vi "Resize Image to a Container 2012 NIVerified.vi"(7 "error in (no error)":errorcluster, 9 "image data":T1, 10 "Path to Image (PNG, JPEG, BMP)":path) -> (0 "error out":errorcluster, 3 "Resized Image":picture)   [LabVIEW 2021, in "Component Tray.lvclass"]
doc: "Demonstrate how to use Base LabVIEW functions and property nodes to manipulate different picture images"
uses:
  Component Tray.lvclass
  <vilib>/picture/picture.llb/imagedata.ctl
panel:
  out "Resized Container":picture
  out "Original":picture
  # "Overview：Demonstrate  how to use Base LabVIEW functions and property nodes to manipulate different picture images\nRequirements:  LabVIEW 2012 or compatible\nInstructions:\n1. Run the VI\n2. Select the location of the image file using the Path to Image control\n3. Run the VI"
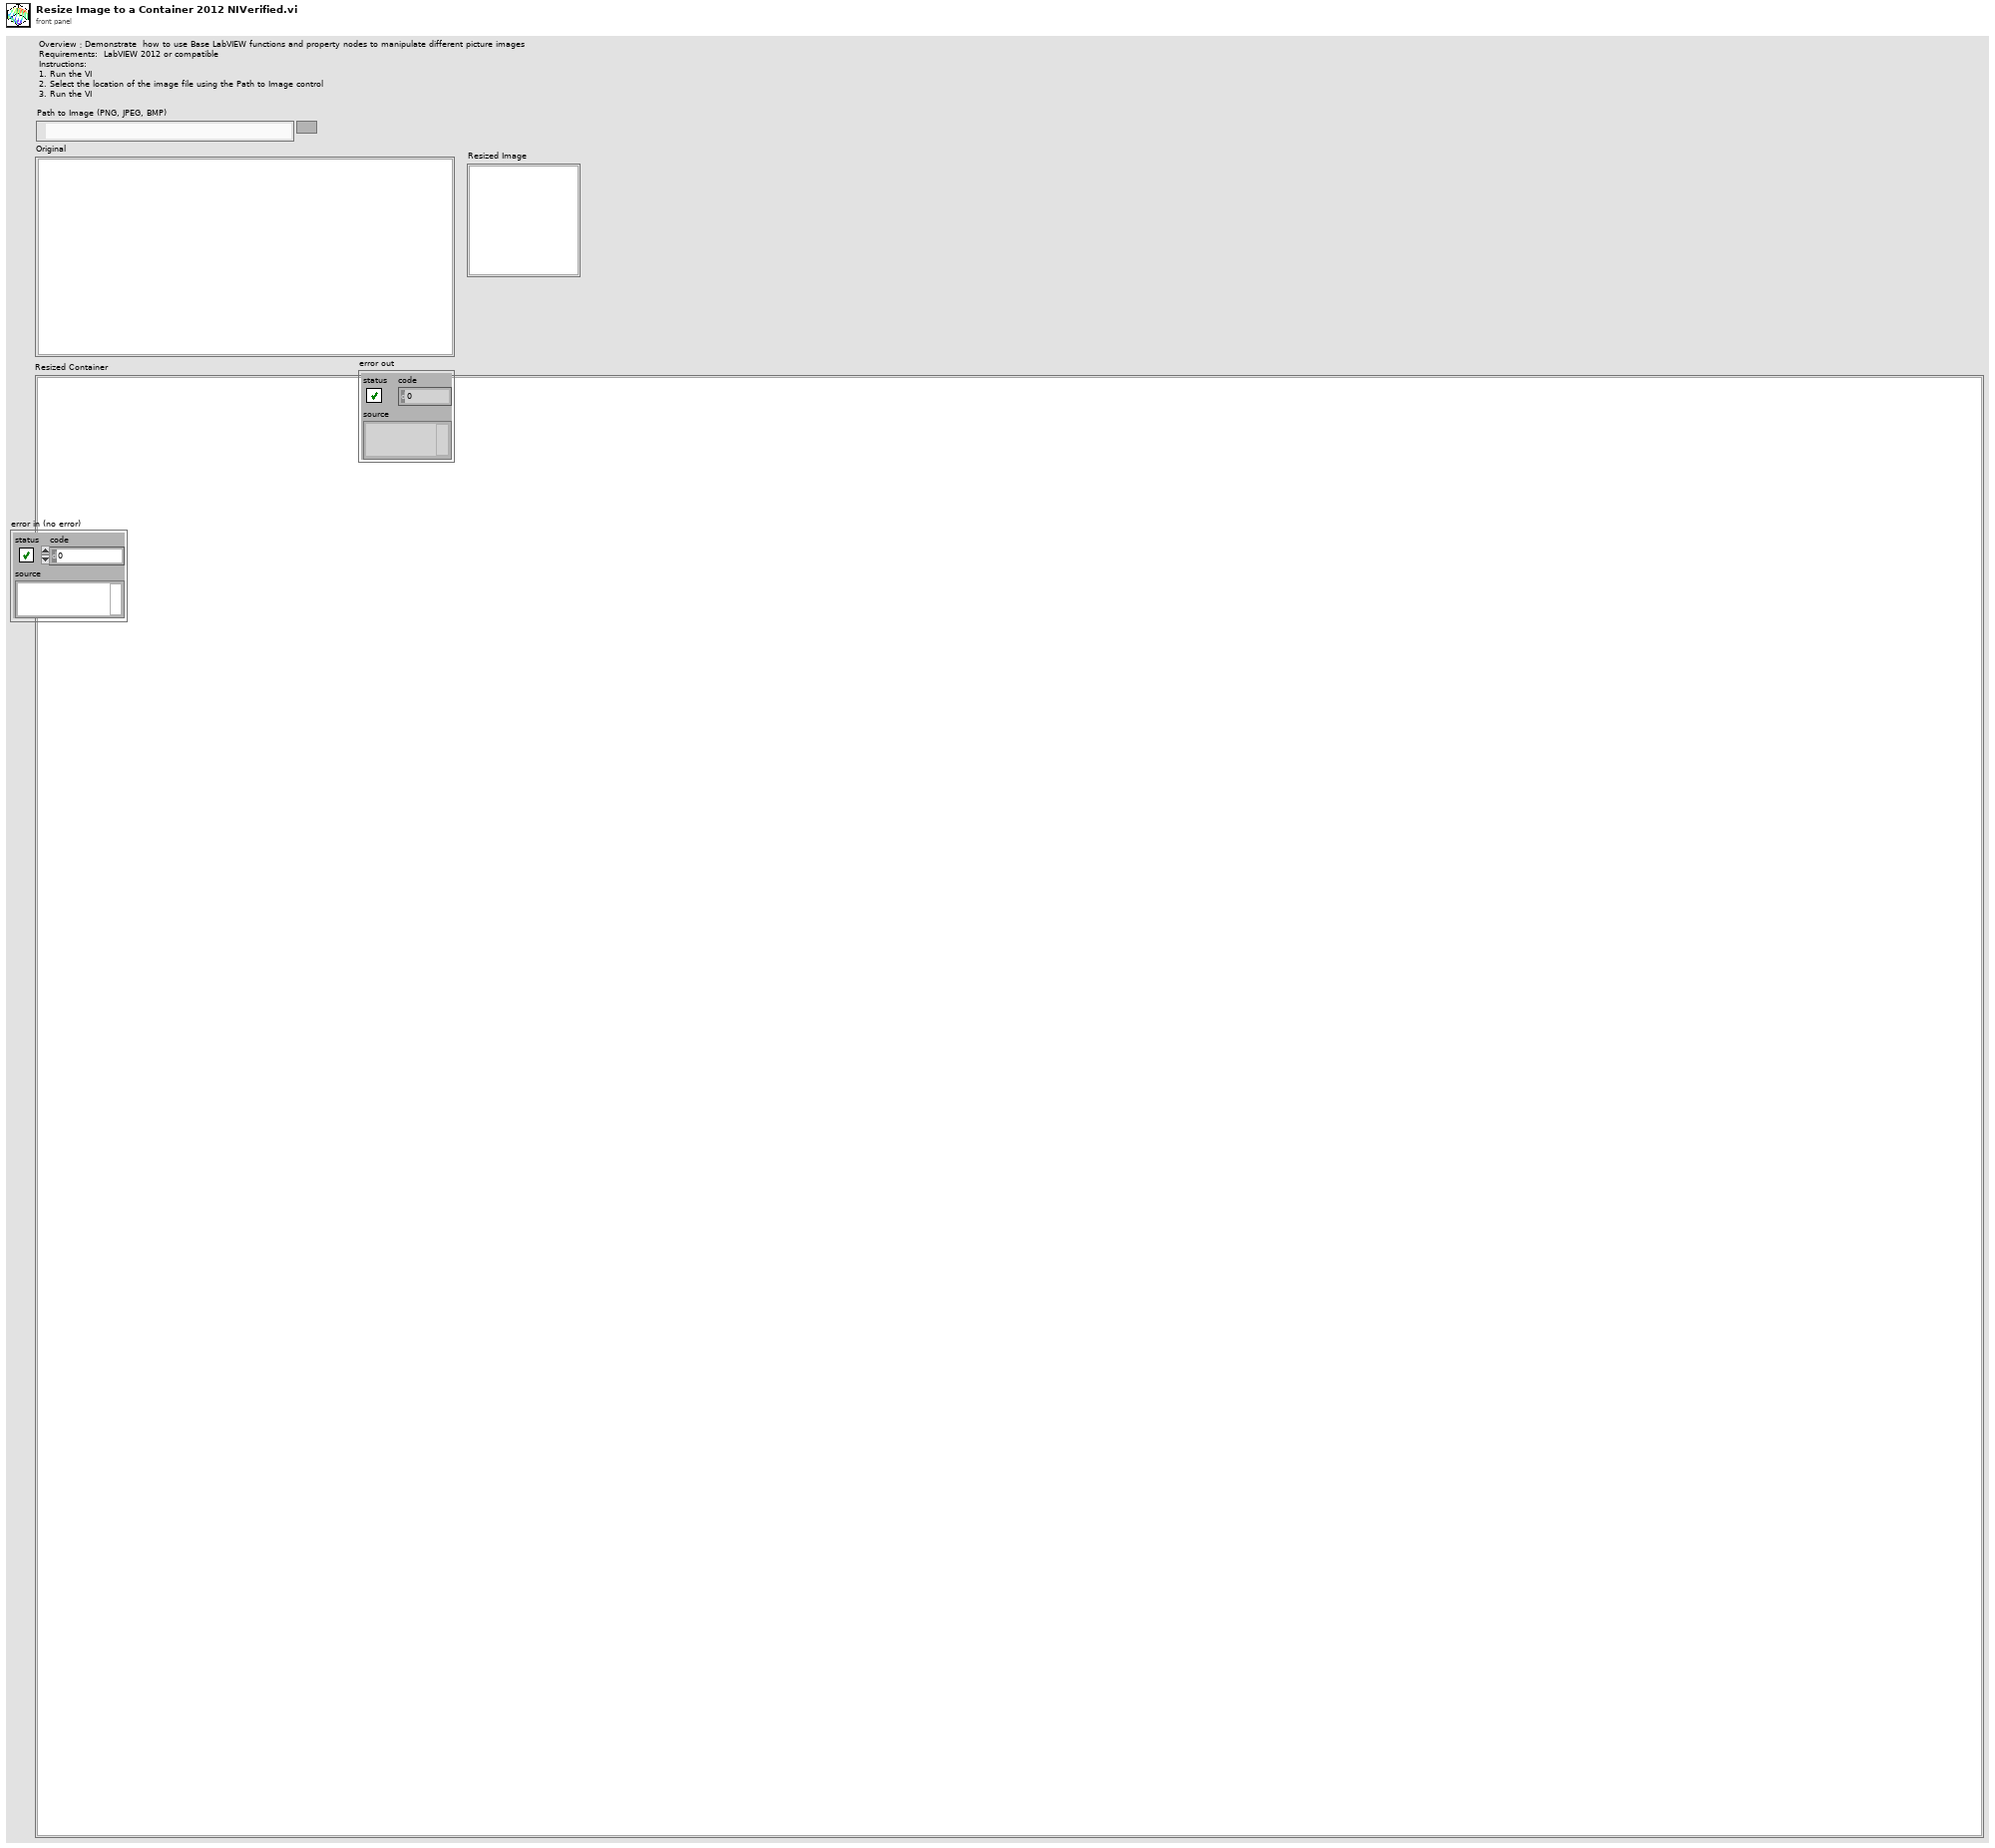
[diagram p1: front panel]
types:
  T1 = typedef "imagedata.ctl" = cluster{"image type":i32, "image depth":i32, "image":u8[], "mask":u8[], "colors":u32[], "Rectangle":cluster{"left":i16, "top":i16, "right":i16, "bottom":i16}}
  T2 = typedef "LVBoundsTypeDef.ctl" = cluster{"Width":u32, "Height":u32}
  T3 = cluster{"left":i16, "top":i16, "right":i16, "bottom":i16}
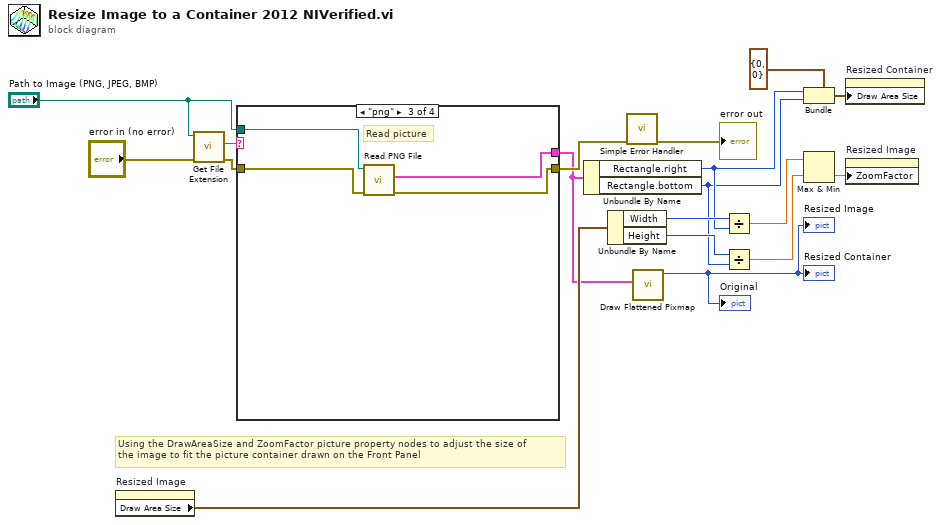
[diagram p0: block diagram]
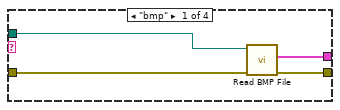
[diagram p2: hidden frame]
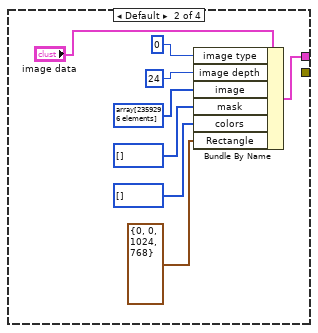
[diagram p3: hidden frame]
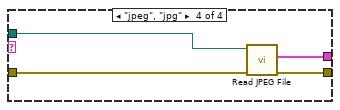
[diagram p4: hidden frame]
diagram:
  # "Using the DrawAreaSize and ZoomFactor picture property nodes to adjust the size of \nthe image to fit the picture container drawn on the Front Panel"
  n1 = property on="Resized Image" class="Pict"() -> ("Draw Area Size"=w18:T2)  [unwired: 2 in, 2 out]
  n2 = call <vilib>:"Get File Extension.vi"("error in (no error)"="error in (no error)", "file"="Path to Image (PNG, JPEG, BMP)") -> ("error out"=w5:errorcluster, "lowercase file extension"=w6:string)  [unwired: 5 in, 3 out]
  n3 = case shown="\"png\"" w6 {
    tunnel: "Path to Image (PNG, JPEG, BMP)" -> [w22 _ w34 w38]
    tunnel: [w21 w23 w33 w37] -> w3
    tunnel: [w20 _ w32 w36] -> w4
    tunnel: w5 -> [w19 _ w31 w35]
    frame "bmp" {
      n4 = call <vilib>:"Read BMP File.vi"("error in (no error)"=w19, "path to BMP file"=w22) -> ("error out"=w20:errorcluster, "image data"=w21:T1)  [unwired: 7 in, 1 out]
    }
    frame Default {
      n5 = Bundle By Name(cluster="image data", "image type"=0, "image depth"=24, "image"=u8[] array[2359296 elements], "mask"=u8[] [], "colors"=u32[] [], "Rectangle"=T3 {"left"=0, "top"=0, "right"=1024, "bottom"=768}) -> (w23:T1)
    }
    frame "png" {
      # "Read picture"
      n6 = call <vilib>:"Read PNG File.vi"("error in (no error)"=w31, "path to PNG file"=w34) -> ("error out"=w32:errorcluster, "image data"=w33:T1)  [unwired: 7 in, 1 out]
    }
    frame "jpeg", "jpg" {
      n7 = call <vilib>:"Read JPEG File.vi"("error in (no error)"=w35, "path to JPEG file"=w38) -> ("error out"=w36:errorcluster, "image data"=w37:T1)  [unwired: 7 in, 1 out]
    }
  }
  n8 = Unbundle By Name(w3) -> ("Rectangle.right"=w12:i16, "Rectangle.bottom"=w11:i16)
  n9 = Unbundle By Name(w18) -> ("Width"=w17:u32, "Height"=w16:u32)
  n10 = call <vilib>:"Simple Error Handler.vi"("error in (no error)"=w4) -> ("error out"=→"error out":errorcluster)  [unwired: 4 in, 4 out]
  n11 = call <vilib>:"Draw Flattened Pixmap.vi"("image data"=w3) -> ("new picture"=→"Resized Image" →"Original" →"Resized Container":picture)  [unwired: 8 in]
  n12 = Divide(x=w17, y=w12) -> (x/y=w15:dbl)
  n13 = Divide(x=w16, y=w11) -> (x/y=w14:dbl)
  n14 = Bundle(cluster=cluster{"Width":u32, "Height":u32} {"Width"=0, "Height"=0} ("Draw Area Size"), "Width"=w12, "Height"=w11) -> (w9:cluster{"Width":u32, "Height":u32})
  n15 = Max & Min(x=w15, y=w14) -> (min(x,y)=w13:dbl)  [unwired: 1 out]
  n16 = property on="Resized Container" class="Pict"("Draw Area Size"=w9) -> ()  [unwired: 2 in, 2 out]
  n17 = property on="Resized Image" class="Pict"("ZoomFactor"=w13) -> ()  [unwired: 2 in, 2 out]
